vi "Subvia Using.vi"() -> ()   [LabVIEW 2022 SP3]
panel:
  in  "stop":bool
  out "Boolean":bool
  in  "Numeric 2":dbl
  in  "Numeric":dbl
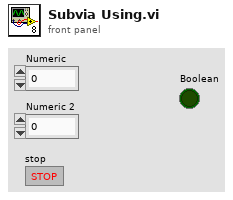
[diagram p1: front panel]
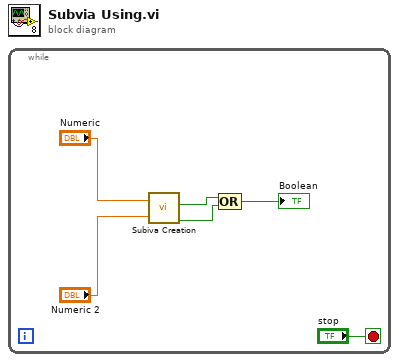
[diagram p0: block diagram]
diagram:
  n1 = while {
    stop <- "stop" stop-if-true
    n2 = call "Subiva Creation.vi"("X"="Numeric", "Y"="Numeric 2") -> ("x > y?"=w3:bool, "x = y?"=w2:bool)  [unwired: 2 out]
    n3 = Compound Arithmetic op=OR(w3, w2) -> (→"Boolean":bool)
  }
